vi "UART Communication.vi"() -> ()   [LabVIEW 2011]
uses:
  <vilib>/Instr/_visa.llb/VISA Configure Serial Port (Instr).vi
  <vilib>/Analysis/NI_AALBase.lvlib
panel:
  in  "Control Box":T1={"Force Divider"=50.0, "Torque Divider"=2000.0}
  out "Loop":u32(knob) scale=0.0..10.0
  out "Force/Torque":dynamicdata(graph)
  in  "Stop":bool
  out "Unbiased DATA":dbl[](array[numeric])
  out "ForceTorque":dbl[](array[numeric])
  out "Bias":dbl[](array[numeric]) format="%#.0f"
  in  "Bias":bool caption="Bias 2"
  in  "UART Communication Block":T2={"baud rate"=115200, "VISA resource name"="COM6", "data bits"=8, "parity"=0, "stop bits"=10, "flow control"=0} {"flow control" items=["None"=0, "XON/XOFF"=1, "RTS/CTS"=2, "DTR/DSR"=4]; "stop bits" items=["1.0"=10, "1.5"=15, "2.0"=20]; "parity" items=["None", "Odd", "Even", "Mark", "Space"]; "data bits" min=5 max=8 step=1}
  in  "Command":bool
  in  "탭 컨트롤":enum32{"T/R ID", "Filter", "Rate"}(tab)=enum."Filter"
  in  "송수신 ID":u16[](array[numeric])
  in  "Cutoff Frequency":u8(ring)=5 items=["None", "500Hz", "300Hz", "200Hz", "150Hz", "100Hz", "50Hz", "40Hz", "30Hz", "20Hz", "10Hz", "5Hz", "3Hz", "2Hz", "1Hz"]
  in  "Filter Type":u16(ring)=1 items=["None", "LowPass Filter"]
  in  "Data Rate":u16(ring) items=["200Hz", "10Hz", "20Hz", "50Hz", "100Hz", "200Hz", "333Hz", "500Hz", "1000Hz"]
  in  "Setting":T3={"필터종류"=0, "속도 ID"=1, "출력 주기"=0, "필터 세부 정보"=0, "송수신 ID"=[]} {"출력 주기" items=["200Hz"=0, "500Hz"=2, "1000Hz"=1]; "속도 ID" items=["1 Mbps"=1, "500Kbps"=2, "250Kbps"=3, "125Kbps"=4, "100Kbps"=5]; "필터종류" items=["None", "Moving Average"]}
  in  "Command":u16(ring) items=["Not yet - Read Product Name", "Not yet - Read Serial Number", "Not yet - Read Firmware Version", "CAN version only - Set ID", "CAN version only - Read ID", "Not yet - Set Baud rate", "Not yet - Read Baud rate", "Set Filter Type", "Not yet - Read Filter Type", "Read F/T 1 sample", "Read F/T", "Stop F/T Out", "Reserved", "Reserved", "Set Output Rate", "Not yet - Read output rate", "Not yet - Set Bias", "Not yet - Read overload count"]
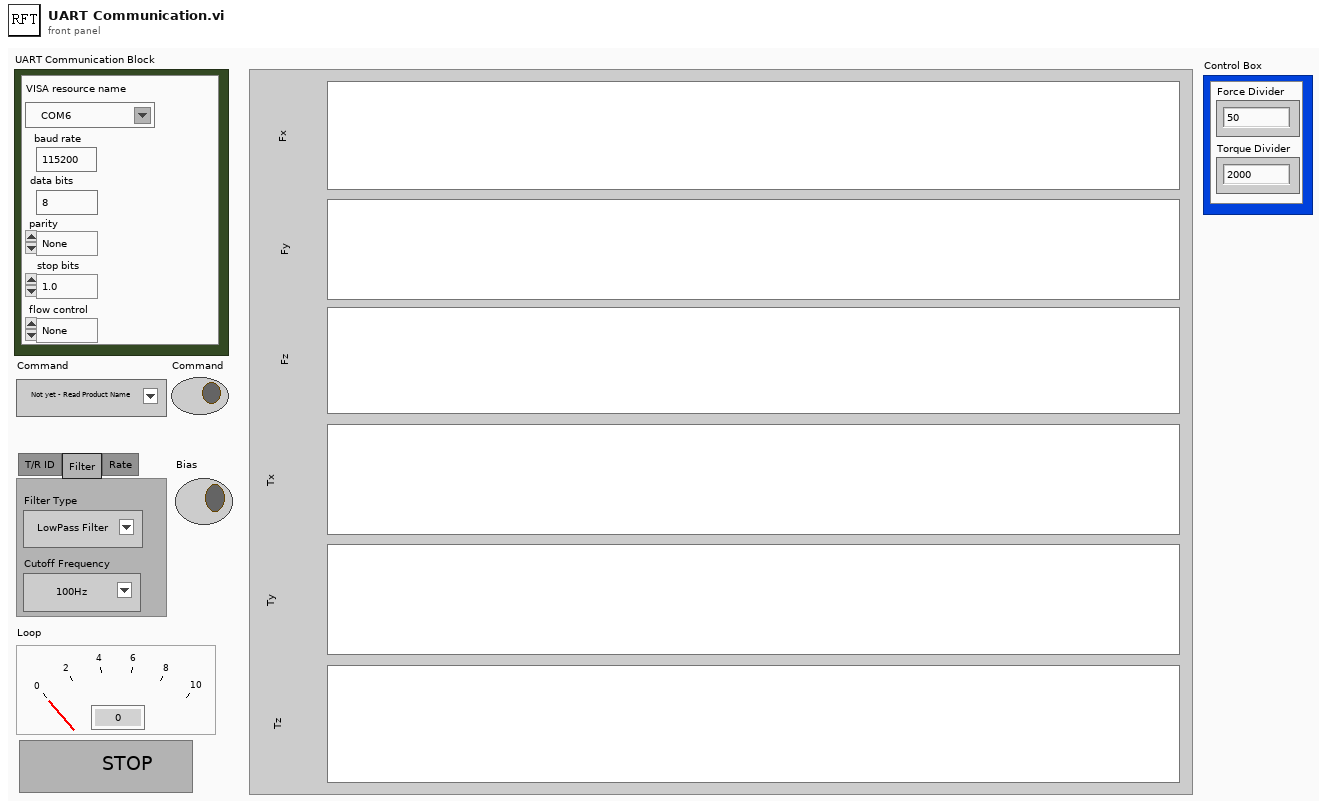
[diagram p1: front panel]
types:
  T1 = cluster{"Force Divider":dbl, "Torque Divider":dbl}
  T2 = cluster{"baud rate":u32, "VISA resource name":refnum<visa-resource-name>, "data bits":u16, "parity":u16, "stop bits":u16, "flow control":u16}
  T3 = cluster{"필터종류":u16, "속도 ID":u16, "출력 주기":u16, "필터 세부 정보":u8, "송수신 ID":u8[]}
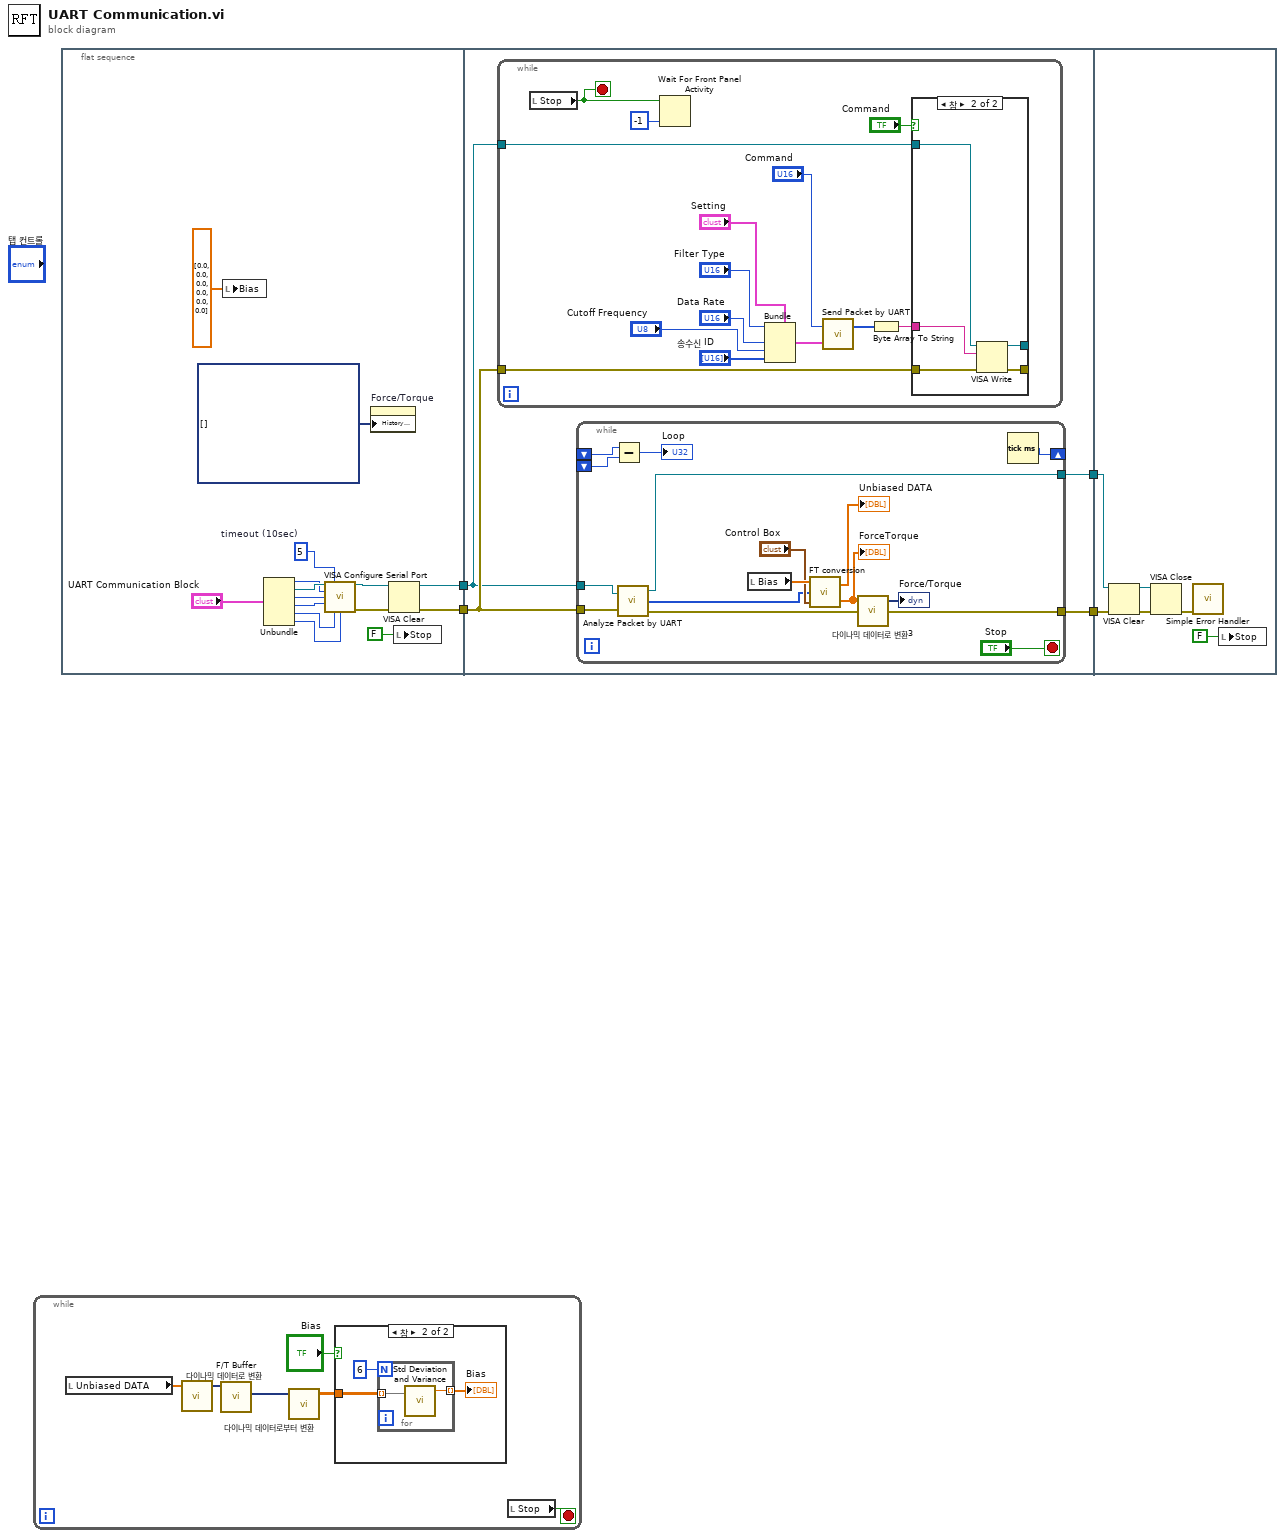
[diagram p0: block diagram]
diagram:
  n1 = while {
    stop <- w10 stop-if-true
    n2 = local read "Unbiased DATA"() -> (w7:dbl[])
    n3 = call "다이나믹 데이터로 변환"("Array"=w7) -> ("Dynamic Data Type"=w8:dynamicdata)  [unwired: 3 in]
    n4 = call "F/T Buffer"("Signals"=w8) -> ("Collected Signals"=w9:dynamicdata)  [unwired: 9 in, 1 out]
    n5 = call "다이나믹 데이터로부터 변환"("Dynamic Data Type"=w9) -> ("Array"=w5:dbl[][])  [unwired: 3 in]
    n6 = case shown="참" "Bias" {
      tunnel: w5 -> [_ w12]
      frame False {
      }
      frame True {
        n7 = for {
          N: 6 -> [_]
          tunnel: w12 -> [w15] mode=indexing
          tunnel: [w14] -> w11 mode=indexing
          n8 = call <vilib>:"Std Deviation and Variance.vi"("X"=w15) -> ("mean"=w14:dbl)  [unwired: 1 in, 2 out]
        }
        "Bias" <- w11
      }
    }
    n9 = local read "Stop"() -> (w10:bool)
  }
  n10 = flat-sequence {
    tunnel: [w16] -> w4
    tunnel: [w17] -> w1
    tunnel: w4 -> [w32]
    tunnel: [w34] -> w3
    tunnel: [w33] -> w2
    tunnel: w1 -> [w31]
    tunnel: w3 -> [w73]
    tunnel: w2 -> [w74]
    frame #0 {
      w23 = u32 5  # timeout (10sec)
      n11 = local write "Bias"(dbl[] [0.0, 0.0, 0.0, 0.0, 0.0, 0.0] ("Bias")) -> ()
      n12 = Unbundle("UART Communication Block") -> ("baud rate"=w25:u32, "VISA resource name"=w26:refnum<visa-resource-name>, "data bits"=w27:u16, "parity"=w28:u16, "stop bits"=w29:u16, "flow control"=w30:u16)
      n13 = call-poly "VISA Configure Serial Port"("VISA resource name"=w26, "timeout (10sec)"=w23, "baud rate (9600)"=w25, "data bits (8)"=w27, "parity (0:none)"=w28, "stop bits (10: 1 bit)"=w29, "flow control (0:none)"=w30) -> ("VISA resource name out"=w19:refnum<visa-resource-name>, "error out"=w18:errorcluster)  [unwired: 2 in, 5 out]
      n14 = property on="Force/Torque" class="WFChart (엄격한)"("History Data"=dynamicdata[] [] ("히스토리 데이터")) -> ()  [unwired: 2 in, 2 out]
      n15 = VISA Clear(VISA resource name=w19, error in (no error)=w18) -> (VISA resource name out=w17:refnum<visa-resource-name>, error out=w16:errorcluster)
      n16 = local write "Stop"(FALSE ("Stop")) -> ()
    }
    frame #1 {
      n17 = while {
        tunnel: w31 -> [w38]
        tunnel: w32 -> [w37]
        stop <- w35 stop-if-true
        n18 = local read "Stop"() -> (w35:bool)
        n19 = Wait For Front Panel Activity(1:-1 ("타임아웃 ms (-1 타임아웃 없음)"), 3:w35) -> ()  [unwired: 1 in, 1 out]
        n20 = Bundle(cluster="Setting", "필터종류"="Filter Type", "출력 주기"="Data Rate", "필터 세부 정보"="Cutoff Frequency", "송수신 ID"="송수신 ID") -> (w42:T3)  [unwired: 1 in]
        n21 = call "Send Packet by UART.vi"("기타 설정"=w42, "Command"="Command") -> ("Packet"=w40:u8[])  [unwired: 1 out]
        n22 = Byte Array To String(unsigned byte array=w40) -> (string=w39:string)
        n23 = case shown="참" "Command" {
          tunnel: [w49 w53] -> _
          tunnel: w38 -> [w50 w55]
          tunnel: w37 -> [w49 w54]
          tunnel: [w50 w52] -> _
          tunnel: w39 -> [_ w51]
          frame False {
          }
          frame True {
            n24 = VISA Write(VISA resource name=w55, write buffer=w51, error in (no error)=w54) -> (VISA resource name out=w52:refnum<visa-resource-name>, error out=w53:errorcluster)  [unwired: 1 out]
          }
        }
      }
      n25 = while {
        tunnel: [w58] -> w34
        tunnel: [w59] -> w33
        shift-right: [w69] -> _
        shift-left: _ -> [w68]
        shift-left: _ -> [w67]
        tunnel: w32 -> [w60]
        tunnel: w31 -> [w61]
        stop <- "Stop" stop-if-true
        n26 = Subtract(x=w68, y=w67) -> (x-y=→"Loop":u32)
        n27 = call "Analyze Packet by UART.vi"("VISA resource name in"=w61, "error in"=w60) -> ("VISA resource name out"=w59:refnum<visa-resource-name>, "Packet"=w56:u8[], "error out"=w58:errorcluster)
        n28 = local read "Bias"() -> (w63:dbl[])
        n29 = call "FT conversion.vi"("Control Box"="Control Box", "Raw Data"=w56, "Bias"=w63) -> ("ForceTorque"=w65:dbl[], "Unbiased DATA"=→"Unbiased DATA":dbl[])
        "ForceTorque" <- w65
        n30 = call "다이나믹 데이터로 변환3"("Array"=w65) -> ("Dynamic Data Type"=→"Force/Torque":dynamicdata)  [unwired: 3 in]
        n31 = Tick Count (ms)() -> (millisecond timer value=w69:u32)
      }
    }
    frame #2 {
      n32 = VISA Clear(VISA resource name=w74, error in (no error)=w73) -> (VISA resource name out=w72:refnum<visa-resource-name>, error out=w71:errorcluster)
      n33 = VISA Close(VISA resource name=w72, error in (no error)=w71) -> (error out=w76:errorcluster)
      n34 = call <vilib>:"Simple Error Handler.vi"("error in (no error)"=w76) -> ()  [unwired: 1 in, 8 out]
      n35 = local write "Stop"(FALSE ("Stop")) -> ()
    }
  }
